vi "Get State (uSMC).vi"(8 "error in (no error)":errorcluster, 9 "SM number":i32, 11 "Visa array in":refnum<visa-resource-name>[](array[refnum])) -> (0 "error out":errorcluster, 1 "State cluster":T1, 3 "Visa array out":refnum<visa-resource-name>[](array[refnum]))   [LabVIEW 2010, in "SignalWriterMH110203USBStepperMotor.lvclass"]
uses:
  SignalWriterMH110203USBStepperMotor.lvclass
  Get State Control (uSMC).ctl
  class_data.vi
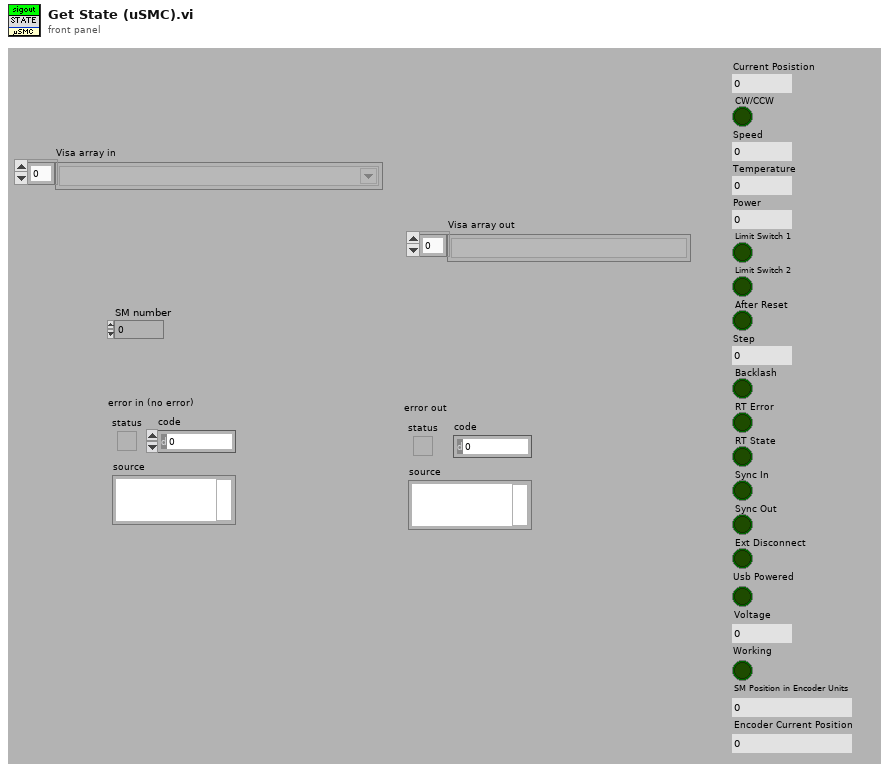
[diagram p1: front panel]
types:
  T1 = typedef "SignalWriterMH110203USBStepperMotor.lvclass/Get State Control (uSMC).ctl" = cluster{"Current Posistion":dbl, "CW/CCW":bool, "Speed":u16, "Temperature":dbl, "Power":u16, "Limit Switch 1":bool, "Limit Switch 2":bool, "After Reset":bool, "Step":u8, "Backlash":bool, "RT Error":bool, "RT State":bool, "Sync In":bool, "Sync Out":bool, "Ext Disconnect":bool, "Usb Powered":bool, "Voltage":dbl, "Working":bool, "SM Position in Encoder Units":i32, "Encoder Current Position":i32}
  T2 = cluster{"Cur Pos Units":dbl, "Set Cur Pos units":dbl, "Lo Limit Units":dbl, "Hi Limit Units":dbl, "Cur Pos Ticks":i32, "Set Cur Pos ticks":i32, "Lo Limit Ticks":i32, "Hi Limit Ticks":i32, "Minimal Value":dbl, "Maximal Value":dbl}[]
  T3 = cluster{"Cur Pos Units":dbl, "Set Cur Pos units":dbl, "Lo Limit Units":dbl, "Hi Limit Units":dbl, "Cur Pos Ticks":i32, "Set Cur Pos ticks":i32, "Lo Limit Ticks":i32, "Hi Limit Ticks":i32, "Minimal Value":dbl, "Maximal Value":dbl}
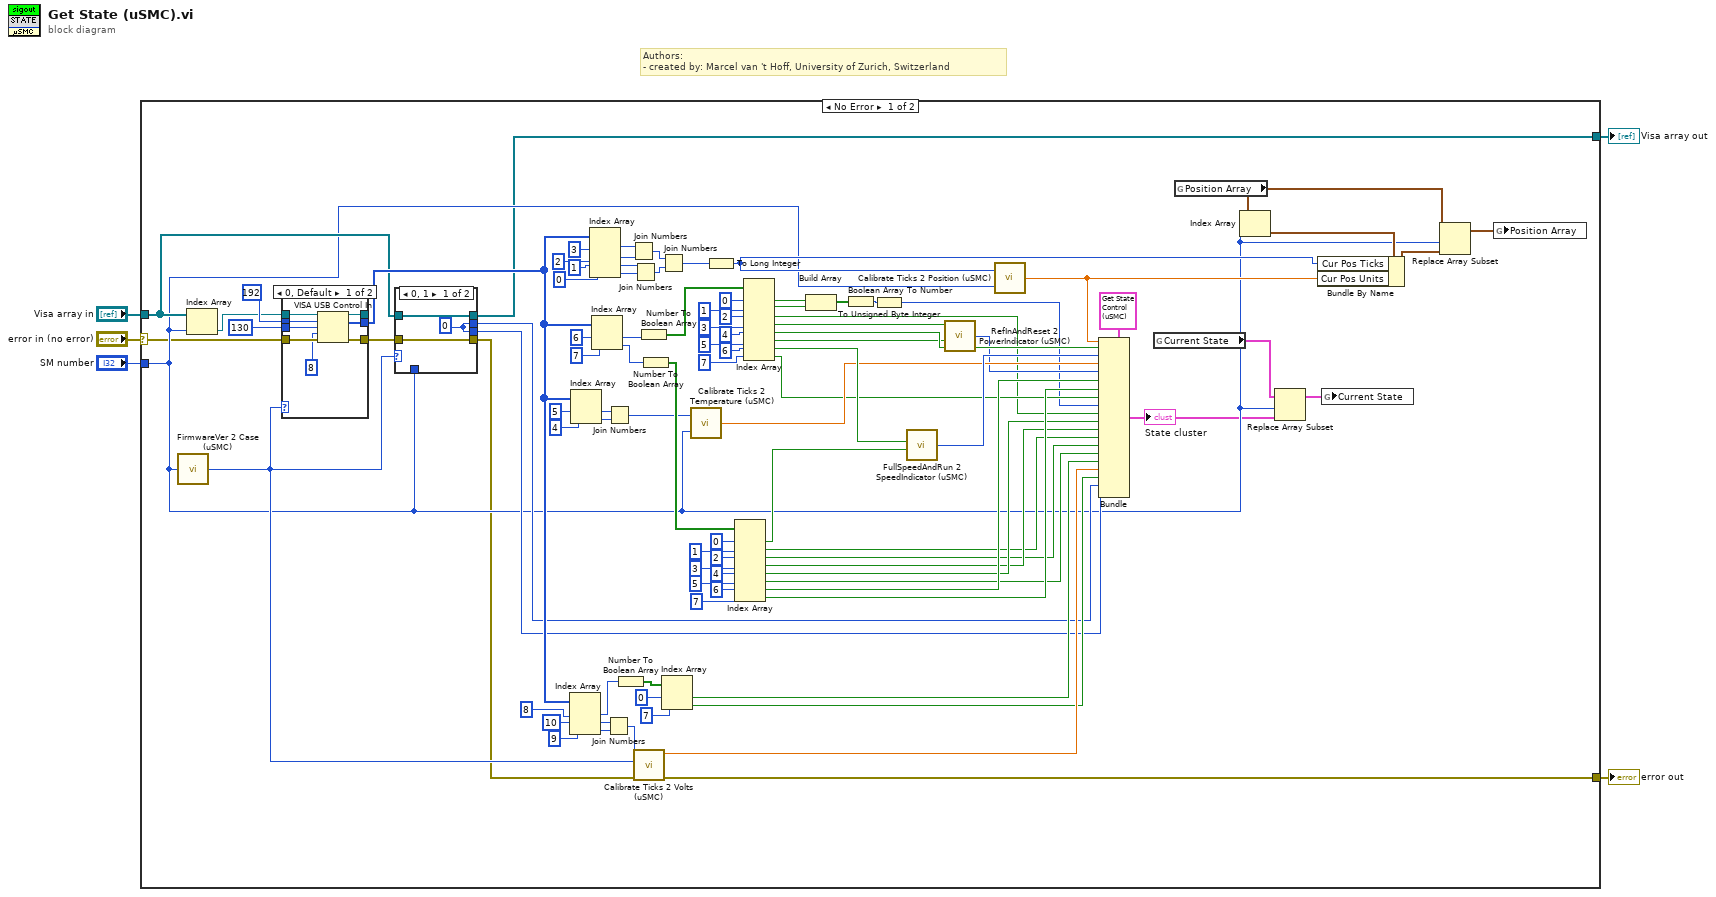
[diagram p0: block diagram]
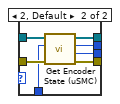
[diagram p2: hidden frame]
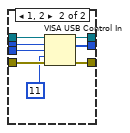
[diagram p3: hidden frame]
diagram:
  # "Authors: \n- created by: Marcel van 't Hoff, University of Zurich, Switzerland"
  n1 = case shown="No Error" "error in (no error)" {
    selector: "error in (no error)" -> [w10 w130]
    tunnel: "Visa array in" -> [w24 w129]
    tunnel: "SM number" -> [w16 _]
    tunnel: [w11 w129] -> w3
    tunnel: [w9 w130] -> w2
    frame No Error {
      n2 = call "FirmwareVer 2 Case (uSMC).vi"("SMindex"=w16) -> ("Case"=w23:i32)
      n3 = Index Array(array=w24, index=w16) -> (element=w59:refnum<visa-resource-name>)
      n4 = case shown="0, Default" w23 {
        tunnel: i16 192 ("request type") -> [w120 w128]
        tunnel: i16 130 ("request") -> [w119 w127]
        tunnel: w10 -> [w118 w126]
        tunnel: [w117 w125] -> w25
        tunnel: [w115 w123] -> w35
        tunnel: w59 -> [w114 w122]
        tunnel: [w113 w121] -> _
        frame 0, Default {
          n5 = VISA USB Control In(0:w114, 5:w120, 7:w119, 9:u16 8 ("length (0)"), 11:w118) -> (4:w113:refnum<visa-resource-name>, 6:w115:u8[], 15:w117:errorcluster)  [unwired: 2 in]
        }
        frame 1, 2 {
          n6 = VISA USB Control In(0:w122, 5:w128, 7:w127, 9:u16 11 ("length (0)"), 11:w126) -> (4:w121:refnum<visa-resource-name>, 6:w123:u8[], 15:w125:errorcluster)  [unwired: 2 in]
        }
      }
      n7 = case shown="0, 1" w23 {
        tunnel: w25 -> [w104 w112]
        tunnel: [w104 w111] -> w8
        tunnel: w24 -> [w105 w110]
        tunnel: [w105 w109] -> w11
        tunnel: w16 -> [_ w108]
        tunnel: [w103 w107] -> w22
        tunnel: [w103 w106] -> w21
        frame 0, 1 {
          w103 = 0 ("Current Position in Encoder Units")
        }
        frame 2, Default {
          n8 = call "Get Encoder State (uSMC).vi"("error in (no error)"=w112, "SMindex"=w108, "Visa array in"=w110) -> ("error out"=w111:errorcluster, "Encoder Current position"=w106:i32, "Current Position in Encoder Units"=w107:i32, "Visa array out"=w109:refnum<visa-resource-name>[])  [unwired: 5 in]
        }
      }
      n9 = Index Array(array=w35, index #1=8 ("index"), index #2=10 ("index"), index #3=9 ("index")) -> (element #1=w33:u8, element #2=w38:u8, element #3=w39:u8)
      n10 = Index Array(array=w35, index #1=5 ("index"), index #2=4 ("index")) -> (element #1=w63:u8, element #2=w62:u8)
      n11 = Index Array(array=w35, index #1=3 ("index"), index #2=2 ("index"), index #3=1 ("index"), index #4=0 ("index")) -> (element #1=w95:u8, element #2=w96:u8, element #3=w94:u8, element #4=w93:u8)
      n12 = Index Array(array=w35, index #1=6 ("index"), index #2=7 ("index")) -> (element #1=w88:u8, element #2=w87:u8)
      n13 = Join Numbers(hi=w38, lo=w39) -> ((hi.lo)=w29:u16)
      n14 = Join Numbers(hi=w63, lo=w62) -> ((hi.lo)=w40:u16)
      n15 = Number To Boolean Array(number=w33) -> (Boolean array=w32:bool[])
      n16 = Join Numbers(hi=w95, lo=w96) -> ((hi.lo)=w92:u16)
      n17 = Join Numbers(hi=w94, lo=w93) -> ((hi.lo)=w91:u16)
      n18 = call "Calibrate Ticks 2 Volts (uSMC).vi"("error in (no error)"=w8, "Case"=w23, "VoltageTicks"=w29) -> ("error out"=w9:errorcluster, "VoltageVolts"=w28:dbl)  [unwired: 7 in]
      n19 = Number To Boolean Array(number=w88) -> (Boolean array=w86:bool[])
      n20 = Number To Boolean Array(number=w87) -> (Boolean array=w66:bool[])
      n21 = Join Numbers(hi=w92, lo=w91) -> ((hi.lo)=w61:u32)
      n22 = Index Array(array=w32, index #1=0 ("index"), index #2=7 ("index")) -> (element #1=w30:bool, element #2=w26:bool)
      n23 = call "Calibrate Ticks 2 Temperature (uSMC).vi"("SMindex"=w16, "temperature (ticks)"=w40) -> ("Temperature (Cels)"=w53:dbl)
      n24 = To Long Integer(number=w61) -> (32bit integer=w19:i32)
      n25 = Index Array(array=w66, index #1=0 ("index"), index #2=1 ("index"), index #3=2 ("index"), index #4=3 ("index"), index #5=4 ("index"), index #6=5 ("index"), index #7=6 ("index"), index #8=7 ("index")) -> (element #1=w57:bool, element #2=w43:bool, element #3=w42:bool, element #4=w44:bool, element #5=w45:bool, element #6=w41:bool, element #7=w51:bool, element #8=w50:bool)
      n26 = Index Array(array=w86, index #1=0 ("index"), index #2=1 ("index"), index #3=2 ("index"), index #4=3 ("index"), index #5=4 ("index"), index #6=5 ("index"), index #7=6 ("index"), index #8=7 ("index")) -> (element #1=w77:bool, element #2=w76:bool, element #3=w46:bool, element #4=w56:bool, element #5=w55:bool, element #6=w48:bool, element #7=w58:bool, element #8=w49:bool)
      n27 = Build Array(w77, w76) -> (w75:bool[])
      n28 = Boolean Array To Number(Boolean array=w75) -> (number=w74:u32)
      n29 = To Unsigned Byte Integer(number=w74) -> (unsigned 8bit integer=w47:u8)
      n30 = call "FullSpeedAndRun 2 SpeedIndicator (uSMC).vi"("run"=w57, "full speed"=w58) -> ("speed"=w54:u16)  [unwired: 4 in]
      n31 = call "RefInAndReset 2 PowerIndicator (uSMC).vi"("Reset"=w48, "RefIn"=w56) -> ("Power"=w52:u16)  [unwired: 4 in]
      n32 = call "Calibrate Ticks 2 Position (uSMC).vi"("array index"=w16, "ticks"=w19) -> ("value"=w18:dbl)
      n33 = Bundle(cluster=T1 {"Current Posistion"=-19.759999999999994, "CW/CCW"=TRUE, "Speed"=0, "Temperature"=24.12109375, "Power"=1, "Limit Switch 1"=FALSE, "Limit Switch 2"=FALSE, "After Reset"=TRUE, "Step"=3, "Backlash"=TRUE, "RT Error"=FALSE, "RT State"=TRUE, "Sync In"=TRUE, "Sync Out"=TRUE, "Ext Disconnect"=FALSE, "Usb Powered"=TRUE, "Voltage"=11.703277587890623, "Working"=TRUE, "SM Position in Encoder Units"=-2147321088, "Encoder Current Position"=-2147321086} ("State cluster"), "Current Posistion"=w18, "CW/CCW"=w55, "Speed"=w54, "Temperature"=w53, "Power"=w52, "Limit Switch 1"=w51, "Limit Switch 2"=w50, "After Reset"=w49, "Step"=w47, "Backlash"=w46, "RT Error"=w45, "RT State"=w44, "Sync In"=w43, "Sync Out"=w42, "Ext Disconnect"=w41, "Usb Powered"=w30, "Voltage"=w28, "Working"=w26, "SM Position in Encoder Units"=w22, "Encoder Current Position"=w21) -> (w7:T1)
      "State cluster" <- w7
      n34 = global read "class_data.vi" "Current State"() -> (w15:T1[])
      n35 = global read "class_data.vi" "Position Array"() -> (w13:T2)
      n36 = Index Array(array=w13, index=w16) -> (element=w20:T3)
      n37 = Replace Array Subset(array=w15, new element=w7, index=w16) -> (w14:T1[])
      n38 = Bundle By Name(cluster=w20, "Cur Pos Ticks"=w19, "Cur Pos Units"=w18) -> (w17:T3)
      n39 = global write "class_data.vi" "Current State"(w14) -> ()
      n40 = Replace Array Subset(array=w13, new element=w17, index=w16) -> (w12:T2)
      n41 = global write "class_data.vi" "Position Array"(w12) -> ()
    }
    frame Error {
    }
  }
  "Visa array out" <- w3
  "error out" <- w2
